vi "PLOTSES.vi"() -> ()   [LabVIEW 2015]
panel:
  out "concatenated string":string
  out "standard error":string
  out "standard output":string
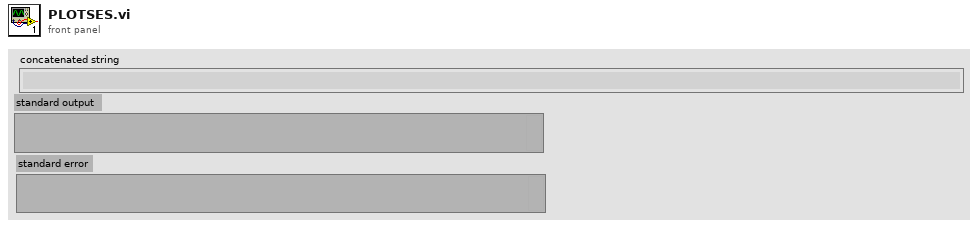
[diagram p1: front panel]
types:
  T1 = enum16{"open", "replace", "create", "open or create", "replace or create", "replace or create with confirmation"}
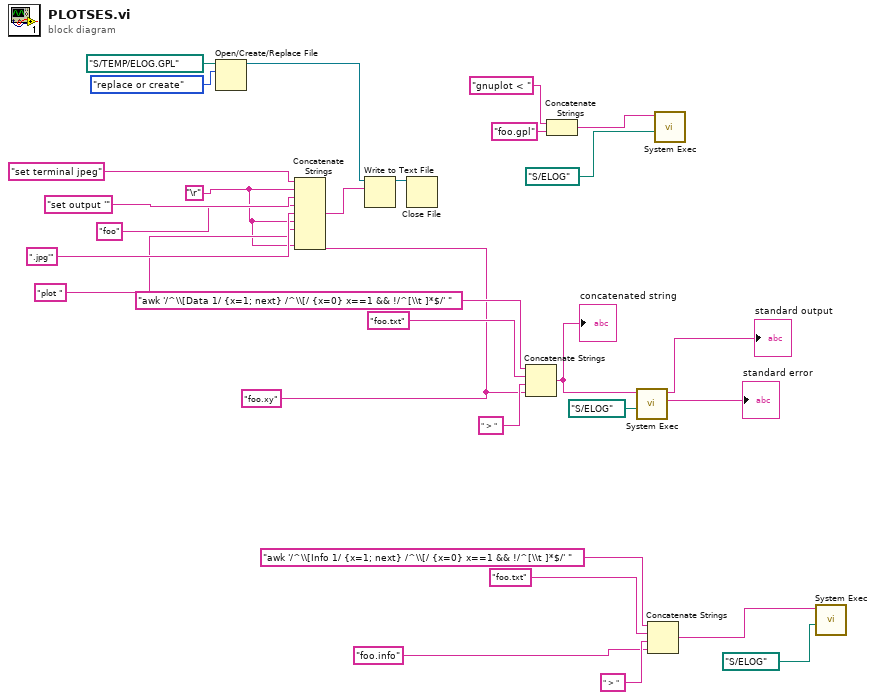
[diagram p0: block diagram]
diagram:
  w11 = "\r"
  w12 = "foo.xy" ("string")
  n1 = Open/Create/Replace File(file path (use dialog)=path "S:/TEMP/ELOG.GPL", operation (0:open)=T1."replace or create") -> (refnum out=w22:refnum<file>)  [unwired: 4 in, 2 out]
  n2 = Concatenate Strings("set terminal jpeg" ("command line"), w11, "set output '" ("command line"), "foo" ("command line"), ".jpg'" ("command line"), w11, "plot " ("command line"), w12, w11) -> (w18:string)
  n3 = Write to Text File(file (use dialog)=w22, text=w18) -> (refnum out=w21:refnum<file>)  [unwired: 2 in, 2 out]
  n4 = Close File(refnum=w21) -> ()  [unwired: 1 in, 2 out]
  n5 = Concatenate Strings("awk '/^\\[Data 1/ {x=1; next} /^\\[/ {x=0} x==1 && !/^[\\t ]*$/' " ("command line"), "foo.txt", " > " ("command line"), w12) -> (w29:string)
  "concatenated string" <- w29
  n6 = Concatenate Strings("gnuplot < " ("command line"), "foo.gpl" ("string")) -> (w8:string)
  n7 = call <vilib>:"System Exec.vi"("working directory"=path "S:/ELOG", "command line"=w29) -> ("standard error"=→"standard error":string, "standard output"=→"standard output":string)  [unwired: 6 in, 2 out]
  n8 = Concatenate Strings("awk '/^\\[Info 1/ {x=1; next} /^\\[/ {x=0} x==1 && !/^[\\t ]*$/' " ("command line"), "foo.txt", " > " ("command line"), "foo.info" ("string")) -> (w1:string)
  n9 = call <vilib>:"System Exec.vi"("working directory"=path "S/ELOG", "command line"=w8) -> ()  [unwired: 6 in, 4 out]
  n10 = call <vilib>:"System Exec.vi"("working directory"=path "S:/ELOG", "command line"=w1) -> ()  [unwired: 6 in, 4 out]
